vi "Galil Terminal IO.vi"(3 "Galil Error In":errorcluster, 4 "Command Input":string, 5 "Reference In":refnum<k7>) -> (0 "Galil Error Out":errorcluster, 1 "Command Output":string, 2 "Reference Out":refnum<k7>)   [LabVIEW 2011]
uses:
  _GlobalVariables&Libraries/ATV Program Global Variables.vi
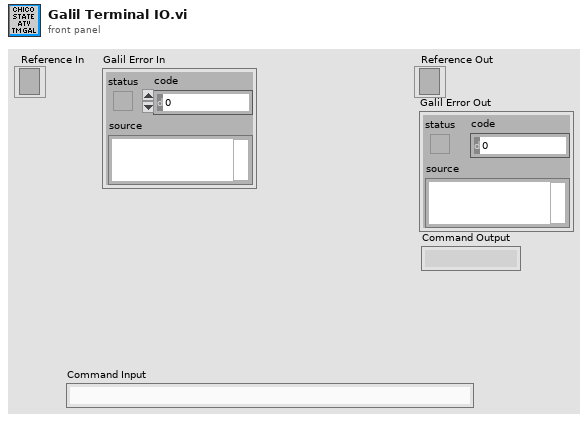
[diagram p1: front panel]
types:
  T1 = cluster{"Drive Value Output String":string, "Steer Value Output String":string, "Error Out":errorcluster, "Initial Encoder Counts":string, "Disable Galil Terminal":bool, "Command Input":string}
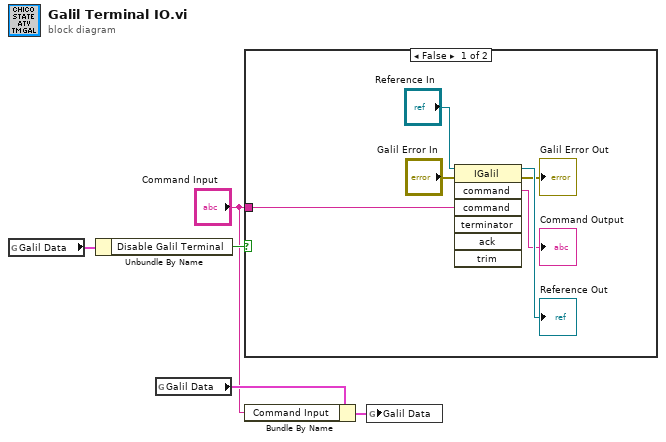
[diagram p0: block diagram]
diagram:
  n1 = global read "ATV Program Global Variables.vi" "Galil Data"() -> (w5:T1)
  n2 = Unbundle By Name(w5) -> ("Disable Galil Terminal"=w4:bool)
  n3 = global read "ATV Program Global Variables.vi" "Galil Data"() -> (w2:T1)
  n4 = case shown="False" w4 {
    tunnel: "Command Input" -> [w6 _]
    frame False {
      n5 = invoke class="IGalil" method="command"(reference="Reference In", error in="Galil Error In", "command"=w6) -> (reference out=→"Reference Out":refnum<k7>, error out=→"Galil Error Out":errorcluster, "command"=→"Command Output":string)  [unwired: 4 in, 4 out]
    }
    frame True {
    }
  }
  n6 = Bundle By Name(cluster=w2, "Command Input"="Command Input") -> (w3:T1)
  n7 = global write "ATV Program Global Variables.vi" "Galil Data"(w3) -> ()
